vi "Coordinate_Trans_.vi"(0 "Traverse Name":string, 1 "Input Position":sgl[](array[numeric])=[0.0, 0.0, 0.0] format="%.2f", 2 "Simulate/Run":T1) -> (3 "X":sgl, 4 "Y":sgl, 5 "Z":sgl, 6 "Error String":string)   [LabVIEW 2021]
uses:
  Controls/User_Specific_mode.ctl
  Controls/Tunnel_Coordinates.ctl
  Globals/Trav_pos_global.vi
  Globals/Extra_Commands_Global.vi
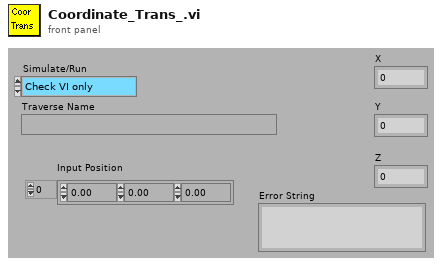
[diagram p1: front panel]
types:
  T1 = typedef "User_Specific_mode.ctl" = enum16{"Check VI only", "Run VI"}
  T2 = typedef "Traverse_cluster.ctl" = cluster{"Start X":sgl, "Start Y":sgl, "Start Z":sgl, "End X":sgl, "End Y":sgl, "End Z":sgl, "nPoints":i32, "Spacing":T3, "Filename":path, "Tunnel Speed":dbl, "Averaging time (mins)":dbl, "Extra Commands":string, "Carrier_1 Q (l/min)":dbl, "Carrier_2 Q (l/min)":dbl, "Trace Gas Concentration (%)":dbl, "Specific Arguments":string, "Comments":string, "Row No":i32, "Row Type Selector":T4, "EstCompl":string, "Row Duration (mins)":dbl, "nValidPoints":i32, "Meas Setup File":string}
  T3 = typedef "Spacing.ctl" = enum16{"Linear", "Log", "Gauss", "Specified", "N/A"}
  T4 = typedef "Multi_run_mode.ctl" = enum16{"Move Traverse Only", "Set Tunnel Speed Only", "Set Source Only", "Set Measurement Conditions", "Single Measurement", "Vertical Profile", "Lateral Profile", "Longitudinal Profile", "Multi-Axis Profile", "Explore Volume", "Auto Calibrate", "Meas Fast FID Bkgnd", "Check Beam Power", "Scanning Valve Measurement", "Run VI Named:", "Set ADAM Ch", "Wait (minutes)", "Send Message", "Synchronize With:", "Fall Back to this Row", "Turn Off Row Repeating", "Traverse 3D Volume", "Blank Row", "Jump to Fall Back Row"}
  T5 = typedef "Tunnel_Coordinates.ctl" = enum16{"Work in Tunnel Coordinates", "Work in Model Coordinates"}
  T6 = enum16{"To Traverse Coordinates", "To User Coordinates"}
  T7 = cluster{"Output Position[0]":sgl, "Output Position[1]":sgl, "Output Position[2]":sgl}
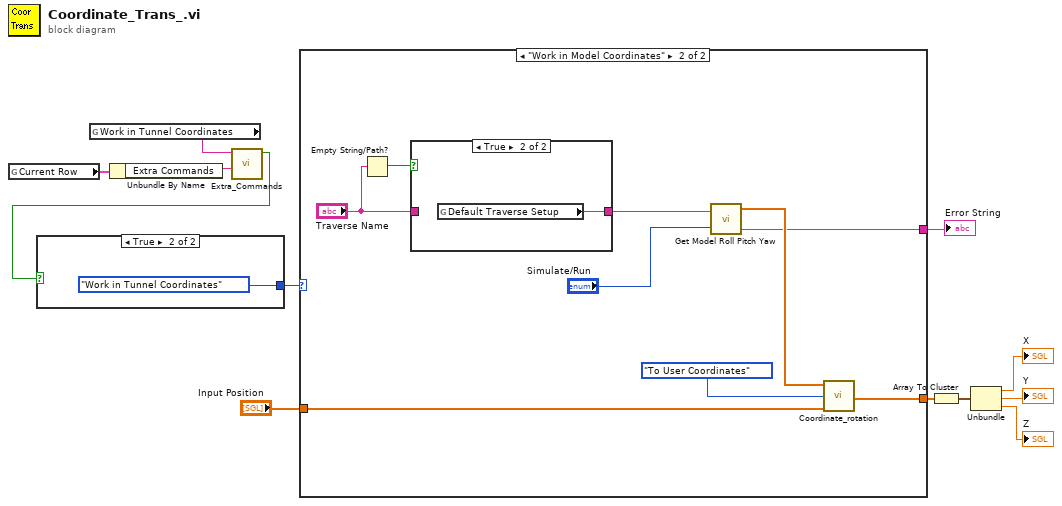
[diagram p0: block diagram]
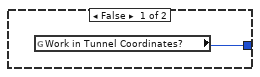
[diagram p2: hidden frame]
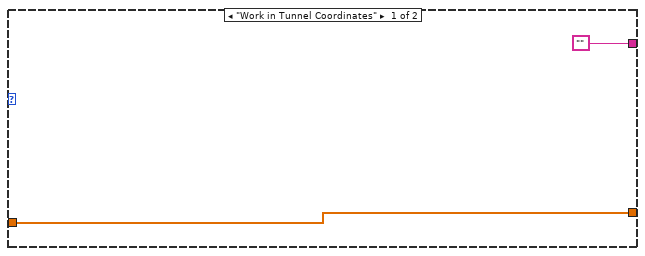
[diagram p3: hidden frame]
diagram:
  n1 = global read "Trav_pos_global.vi" "Current Row"() -> (w4:T2)
  n2 = global read "Extra_Commands_Global.vi" "Work in Tunnel Coordinates"() -> (w6:string)
  n3 = Unbundle By Name(w4) -> ("Extra Commands"=w5:string)
  n4 = call "Extra_Commands.vi"("String to Search"=w5, "Command"=w6) -> ("Command Found"=w3:bool)  [unwired: 1 in, 4 out]
  n5 = case shown="True" w3 {
    tunnel: [w13 Tunnel_Coordinates."Work in Tunnel Coordinates" ("Work in Tunnel Coordinates?")] -> w2
    frame False {
      n6 = global read "Trav_pos_global.vi" "Work in Tunnel Coordinates?"() -> (w13:T5)
    }
    frame True {
    }
  }
  n7 = case shown="\"Work in Model Coordinates\"" w2 {
    tunnel: [w16 w23] -> w10
    tunnel: "Input Position" -> [w16 w24]
    tunnel: ["" w17] -> w1
    frame "Work in Tunnel Coordinates" {
    }
    frame "Work in Model Coordinates" {
      n8 = Empty String/Path?(string/path="Traverse Name") -> (empty?=w22:bool)
      n9 = case shown="True" w22 {
        tunnel: [w26 w27] -> w20
        tunnel: "Traverse Name" -> [w26 _]
        frame False {
        }
        frame True {
          n10 = global read "Trav_pos_global.vi" "Default Traverse Setup"() -> (w27:string)
        }
      }
      n11 = call "Get Model Roll Pitch Yaw.vi"("Traverse Name"=w20, "Mode"="Simulate/Run") -> ("Model:    Roll        Pitch         Yaw  (deg)"=w18:sgl[], "Error String"=w17:string)  [unwired: 1 in]
      n12 = call "Coordinate_rotation.vi"("Roll-Pitch-Yaw"=w18, "Input Position"=w24, "Mode"=T6."To User Coordinates") -> ("Output Position"=w23:sgl[])  [unwired: 2 in, 1 out]
    }
  }
  "Error String" <- w1
  n13 = Array To Cluster(array=w10) -> (cluster=w11:T7)
  n14 = Unbundle(w11) -> ("Output Position[0]"=→"X":sgl, "Output Position[1]"=→"Y":sgl, "Output Position[2]"=→"Z":sgl)
